vi "IDS_adjustment_getContrastInPermill.vi"(0 "deviceHandle":i32, 5 "axisNumber":i32, 11 "error in (no error)":errorcluster) -> (4 "deviceHandle out":i32, 6 "contrast out":i32, 8 "mixContrast out":i32, 10 "baseline out":i32, 15 "error out":errorcluster)   [LabVIEW 2016]
doc: "int IDS_DLL IDS_adjustment_getContrastInPermill(int axisNumber, int32_t * contrast, int32_t * baseline, int32_t* mixContrast);"
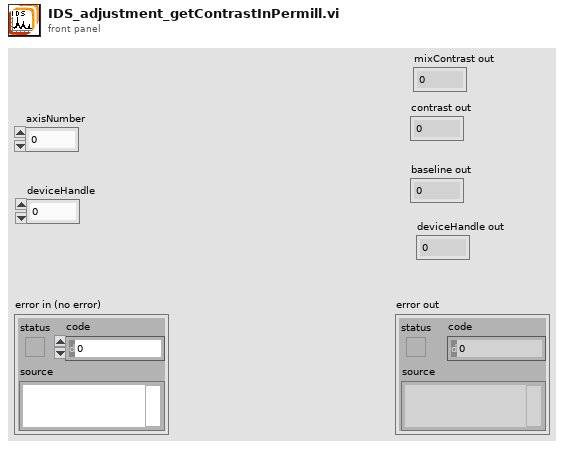
[diagram p1: front panel]
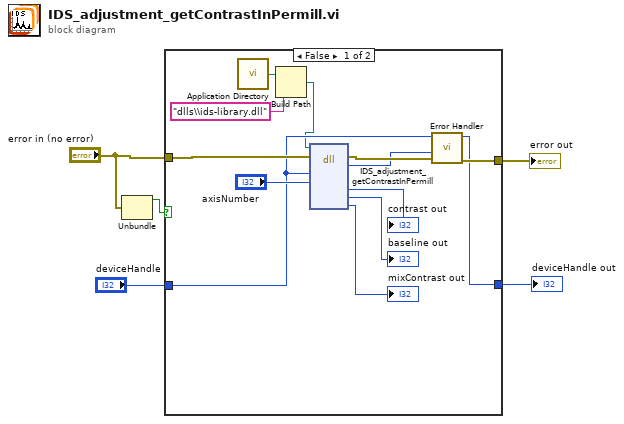
[diagram p0: block diagram]
diagram:
  n1 = Unbundle("error in (no error)") -> ("status"=w1:bool)  [unwired: 2 out]
  n2 = case shown="False" w1 {
    tunnel: [w18 w20] -> w5
    tunnel: "error in (no error)" -> [w16 w20]
    tunnel: "deviceHandle" -> [w10 w19]
    tunnel: [w17 w19] -> w3
    frame False {
      n3 = call <vilib>:"Application Directory.vi"() -> ("Application Directory"=w7:path)
      n4 = Build Path(base path=w7, name or relative path="dlls\\ids-library.dll" ("ipAddress")) -> (appended path=w6:path)
      n5 = dll-call lib="C:/Users/matheus/Desktop/LabVIEW_Draft_V1.6.0/dlls/ids-library.*" fn="IDS_adjustment_getContrastInPermill"(path in=w6, error in=w16, "deviceHandle"=w10, "axisNumber"="axisNumber") -> (error out=w11:errorcluster, "return type"=w9:i32, "contrast"=→"contrast out":i32, "baseline"=→"baseline out":i32, "mixContrast"=→"mixContrast out":i32)  [unwired: 6 in, 1 out]
      n6 = call "Error Handler.vi"("error in (no error)"=w11, "error code"=w9, "deviceHandle"=w10) -> ("error out"=w18:errorcluster, "deviceHandle Out"=w17:i32)  [unwired: 7 in]
    }
    frame True {
    }
  }
  "error out" <- w5
  "deviceHandle out" <- w3
